vi "Evaluate Tx Generic Start - Stop.vi"(10 "current":bool, 11 "last":bool) -> (3 "tx generic command":T1)   [LabVIEW 2020]
uses:
  tx_generic_command.ctl
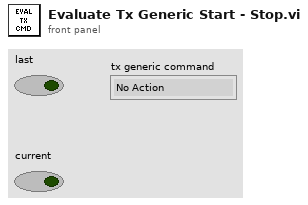
[diagram p1: front panel]
types:
  T1 = typedef "tx_generic_command.ctl" = enum16{"No Action", "Start", "Stop"}
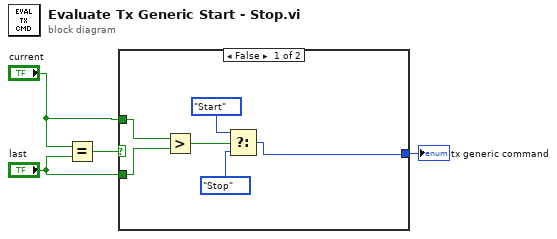
[diagram p0: block diagram]
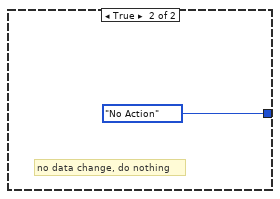
[diagram p2: hidden frame]
diagram:
  n1 = Equal?(x="current", y="last") -> (x = y?=w4:bool)
  n2 = case shown="False" w4 {
    tunnel: [w5 tx_generic_command."No Action"] -> w3
    tunnel: "last" -> [w9 _]
    tunnel: "current" -> [w10 _]
    frame False {
      n3 = Greater?(x=w10, y=w9) -> (0:w8:bool)
      n4 = Select(t=tx_generic_command."Start", s=w8, f=tx_generic_command."Stop") -> (s? t:f=w5:T1)
    }
    frame True {
      # "no data change, do nothing"
    }
  }
  "tx generic command" <- w3
